vi "ChipKit Analog Read Pin.vi"() -> ()   [LabVIEW 2011, in "LabVIEW Interface for ChipKit.lvlib"]
doc: "An example that reads a user selectable analog input pin on the Arduino."
uses:
  vi.lib/LabVIEW Interface for ChipKit/LabVIEW Interface for ChipKit.lvlib
  vi.lib/LabVIEW Interface for ChipKit/Private/Type Defs/Analog Pin.ctl
panel:
  in  "VISA resource name":refnum<visa-resource-name>
  in  "Analog Pin":T1
  in  "Stop":bool
  out "Voltage":dbl(knob) scale=0.0..5.0
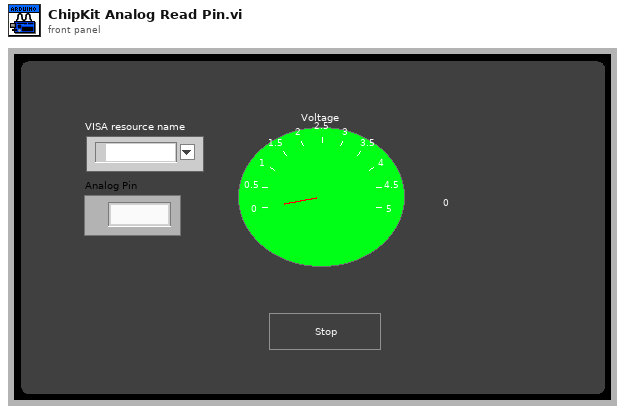
[diagram p1: front panel]
types:
  T1 = typedef "LabVIEW Interface for ChipKit.lvlib/Analog Pin.ctl" = enum8{"AI_0", "AI_1", "AI_2", "AI_3", "AI_4", "AI_5", "AI_6", "AI_7", "AI_8", "AI_9", "AI_10", "AI_11", "AI_12", "AI_13", "AI_14", "AI_15"}
  T2 = typedef "LabVIEW Interface for ChipKit.lvlib/Chipkit Resource.ctl" = cluster{"VISA resource":refnum<visa-resource-name>, "Board Type":T3, "Connection Type":enum8{"USB / Serial"}, "Bytes Per Packet (15)":u8}
  T3 = typedef "LabVIEW Interface for ChipKit.lvlib/Board Type.ctl" = enum16{"Arduino Uno", "Dimuelanove w/Atmega 328", "Mega 2560", "Chipkit Uno32", "Chipkit Max32"}
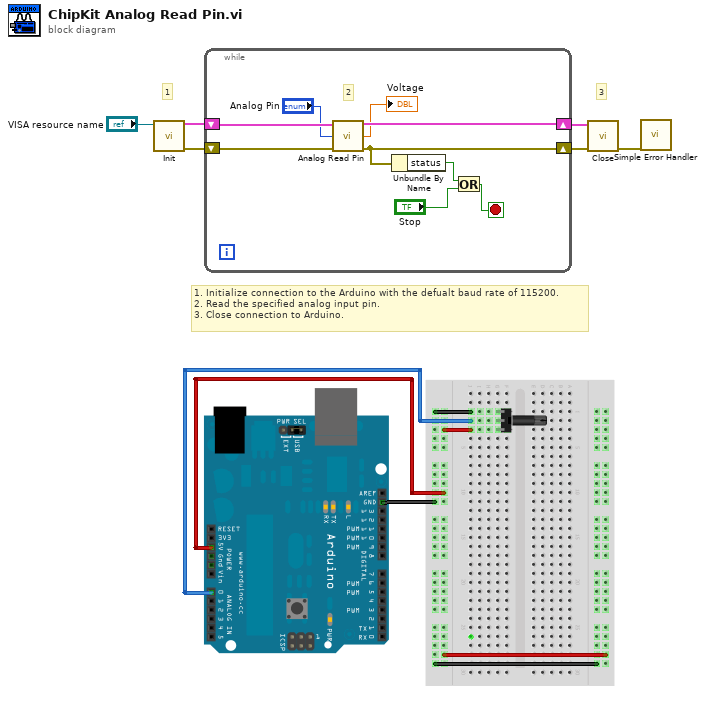
[diagram p0: block diagram]
diagram:
  # "1. Initialize connection to the Arduino with the defualt baud rate of 115200.\n2. Read the specified analog input pin.\n3. Close connection to Arduino."
  # "3"
  # "1"
  n1 = call "Init.vi"("VISA resource"="VISA resource name") -> ("Arduino Resource"=w6:T2, "error out"=w3:errorcluster)  [unwired: 17 in]
  n2 = while {
    shift-right: [w15] -> w5
    shift-left: w6 -> [w9]
    shift-right: [w13] -> w4
    shift-left: w3 -> [w8]
    stop <- w12 stop-if-true
    # "2"
    n3 = call "Analog Read Pin.vi"("Arduino Resource"=w9, "Analog Pin"="Analog Pin", "error in"=w8) -> ("Arduino Resource"=w15:T2, "Voltage"=→"Voltage":dbl, "error out"=w13:errorcluster)  [unwired: 10 in]
    n4 = Unbundle By Name(w13) -> ("status"=w11:bool)
    n5 = Or(x=w11, y="Stop") -> (x .or. y?=w12:bool)
  }
  n6 = call "Close.vi"("Arduino Resource"=w5, "error in"=w4) -> ("error out"=w2:errorcluster)  [unwired: 13 in]
  n7 = call <vilib>:"Simple Error Handler.vi"("error in (no error)"=w2) -> ()  [unwired: 4 in, 5 out]
